vi "Version.vi"(8 "error in (no error)":errorcluster) -> (0 "error out":errorcluster, 2 "version":string)   [LabVIEW 2020, in "lvzstd.lvlib"]
uses:
  lvzstd.lvlib
  Private/Path FGV.vi
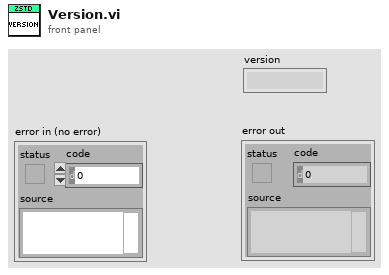
[diagram p1: front panel]
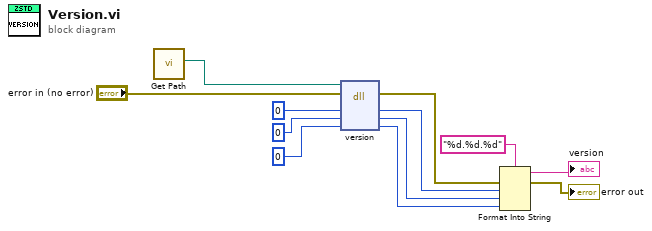
[diagram p0: block diagram]
diagram:
  n1 = call "Get Path.vi"() -> ("Library Path"=w2:path)  [unwired: 10 in, 1 out]
  n2 = dll-call lib="?" fn="version"(path in=w2, error in="error in (no error)", "major"=0, "minor"=0 ("major"), "patch"=0 ("major")) -> (error out=w5:errorcluster, "major"=w9:i32, "minor"=w8:i32, "patch"=w7:i32)  [unwired: 2 in, 1 out]
  n3 = Format Into String(format string="%d.%d.%d", error in=w5, w9, w8, w7) -> (resulting string=→"version":string, error out=→"error out":errorcluster)  [unwired: 1 in]
